vi "SPI Engine. Get Commands from DownStream.vi"(6 "Ready for Output":bool, 8 "error in":errorcluster, 11 "Private Data In":T2={"DLU To SPI Engine Data FIFO"="DLU To SPI Engine Data", "SPI Engine to DLU Data FIFO"="SPI Engine to DLU Data", "Data to SPI Engine (Cache) Register"="Data to SPI Engine (Cache)", "SPI PHY Settings to SPI Engine (Cahche) Register"="SPI PHY Settings to SPI Engine (Cache)"}) -> (0 "error out":errorcluster, 1 "Output Valid":bool, 2 "SPI Transaction Packet":T1, 3 "Private Data Out":T2={"DLU To SPI Engine Data FIFO"="DLU To SPI Engine Data", "SPI Engine to DLU Data FIFO"="SPI Engine to DLU Data", "Data to SPI Engine (Cache) Register"="Data to SPI Engine (Cache)", "SPI PHY Settings to SPI Engine (Cahche) Register"="SPI PHY Settings to SPI Engine (Cache)"}, 5 "Start Strobe":bool)   [LabVIEW 2014]
uses:
  Controls/Internal Data (SPI API).ctl
  Controls/SPI Transaction Packet.ctl
  Controls/SPE Engine. Receiver States.ctl
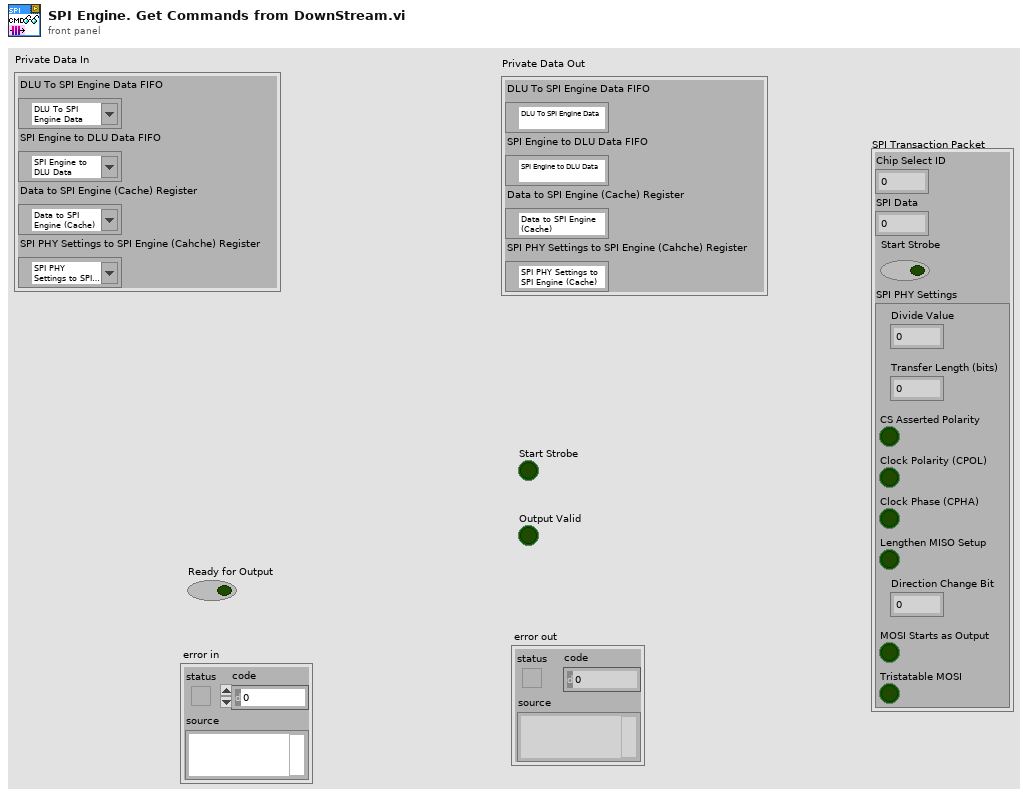
[diagram p1: front panel]
types:
  T1 = typedef "SPI Transaction Packet.ctl" = cluster{"Chip Select ID":u8, "SPI Data":u64, "Start Strobe":bool, "SPI PHY Settings":cluster{"Divide Value":u8, "Transfer Length (bits)":u8, "CS Asserted Polarity":bool, "Clock Polarity (CPOL)":bool, "Clock Phase (CPHA)":bool, "Lengthen MISO Setup":bool, "Direction Change Bit":u8, "MOSI Starts as Output":bool, "Tristatable MOSI":bool}}
  T2 = typedef "Internal Data (SPI API).ctl" = cluster{"DLU To SPI Engine Data FIFO":refnum<k21>, "SPI Engine to DLU Data FIFO":refnum<k21>, "Data to SPI Engine (Cache) Register":refnum<k21>, "SPI PHY Settings to SPI Engine (Cahche) Register":refnum<k21>}
  T3 = typedef "SPE Engine. Receiver States.ctl" = enum16{"Wait for Start Command", "Deassert Start Probe"}
  T4 = cluster{"Chip Select ID":u8, "SPI Data":u64, "SPI PHY Settings":cluster{"Divide Value":u8, "Transfer Length (bits)":u8, "CS Asserted Polarity":bool, "Clock Polarity (CPOL)":bool, "Clock Phase (CPHA)":bool, "Lengthen MISO Setup":bool, "Direction Change Bit":u8, "MOSI Starts as Output":bool, "Tristatable MOSI":bool}}
  T5 = cluster{"Divide Value":u8, "Transfer Length (bits)":u8, "CS Asserted Polarity":bool, "Clock Polarity (CPOL)":bool, "Clock Phase (CPHA)":bool, "Lengthen MISO Setup":bool, "Direction Change Bit":u8, "MOSI Starts as Output":bool, "Tristatable MOSI":bool}
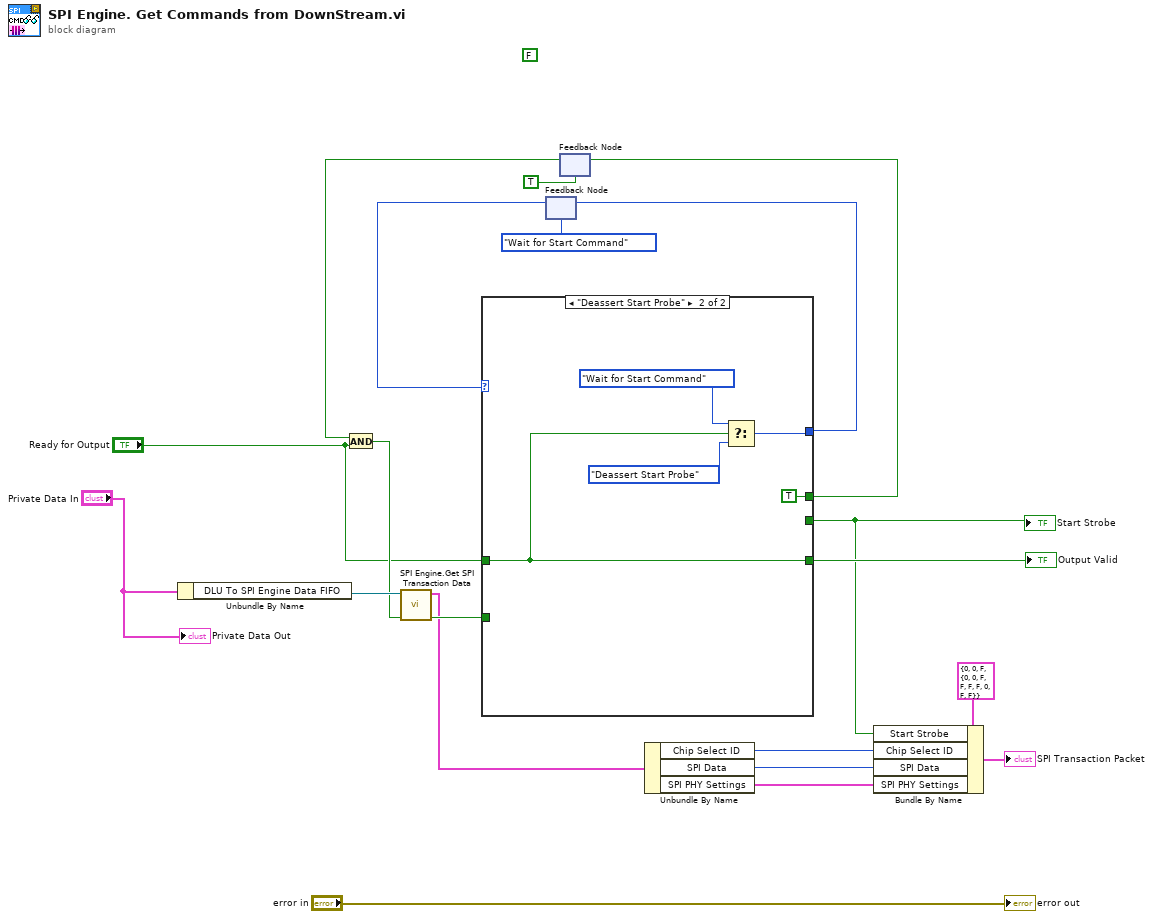
[diagram p0: block diagram]
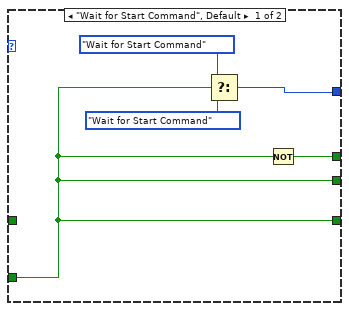
[diagram p2: hidden frame]
diagram:
  (unwired) FALSE
  n1 = Unbundle By Name("Private Data In") -> ("DLU To SPI Engine Data FIFO"=w13:refnum<k21>)
  n2 = feedback #1(SPE_Engine._Receiver_States."Wait for Start Command") -> (w18:T3)
  n3 = feedback #2(TRUE) -> (w15:bool)
  n4 = And(x=w15, y="Ready for Output") -> (x .and. y?=w12:bool)
  n5 = call "SPI Engine.Get SPI Transaction Data.vi"("Get New Data"=w12, "DLU To SPI Engine Data FIFO"=w13) -> ("Output Valid"=w11:bool, "SPI Transaction Data"=w7:T4)  [unwired: 8 in]
  n6 = case shown="\"Deassert Start Probe\"" w18 {
    tunnel: [w23 w26] -> w17
    tunnel: [w22 TRUE] -> w16
    tunnel: w11 -> [w21 _]
    tunnel: [w21 _] -> w3
    tunnel: [w21 w28] -> w10
    tunnel: "Ready for Output" -> [_ w28]
    frame "Wait for Start Command", Default {
      n7 = Select(t=SPE_Engine._Receiver_States."Wait for Start Command", s=w21, f=SPE_Engine._Receiver_States."Wait for Start Command") -> (s? t:f=w23:T3)
      n8 = Not(x=w21) -> (.not. x?=w22:bool)
    }
    frame "Deassert Start Probe" {
      n9 = Select(t=SPE_Engine._Receiver_States."Wait for Start Command", s=w28, f=SPE_Engine._Receiver_States."Deassert Start Probe") -> (s? t:f=w26:T3)
    }
  }
  "Start Strobe" <- w3
  "Output Valid" <- w10
  n10 = feedback-in #1(w17) -> ()
  n11 = feedback-in #2(w16) -> ()
  n12 = Unbundle By Name(w7) -> ("Chip Select ID"=w6:u8, "SPI Data"=w5:u64, "SPI PHY Settings"=w4:T5)
  n13 = Bundle By Name(cluster=T1 {"Chip Select ID"=0, "SPI Data"=0, "Start Strobe"=FALSE, "SPI PHY Settings"={"Divide Value"=0, "Transfer Length (bits)"=0, "CS Asserted Polarity"=FALSE, "Clock Polarity (CPOL)"=FALSE, "Clock Phase (CPHA)"=FALSE, "Lengthen MISO Setup"=FALSE, "Direction Change Bit"=0, "MOSI Starts as Output"=FALSE, "Tristatable MOSI"=FALSE}} ("SPI Transaction Packet"), "Start Strobe"=w3, "Chip Select ID"=w6, "SPI Data"=w5, "SPI PHY Settings"=w4) -> (→"SPI Transaction Packet":T1)
  "Private Data Out" <- "Private Data In"
  "error out" <- "error in"
